vi "StrcatString.vi"() -> ()   [LabVIEW 2012]
uses:
  demo dll.dll
panel:
  out "目标字符串":string
  in  "源字符串2":string
  in  "源字符串1":string
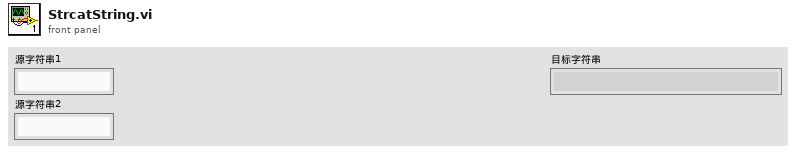
[diagram p1: front panel]
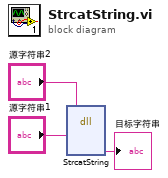
[diagram p0: block diagram]
diagram:
  n1 = dll-call lib="C:/Users/Administrator/Documents/National Instruments/CVI/cvibuild.demo dll/Debug/demo dll.dll" fn="StrcatString"("源字符串1"="源字符串1", "源字符串2"="源字符串2") -> ("目标字符串"=→"目标字符串":string)  [unwired: 7 in, 2 out]
